vi "System-LoadCalibration.vi"   [LabVIEW 2016, in "DSI-RT.lvlib"]
uses:
  DSI-RT.lvlib
  <vilib>/addons/Software Calibration Management/xSCM/CalPoint-Load Calibration.vi
  <vilib>/addons/Software Calibration Management/xSCM/CalPoint-Calibration File Path.vi
  <vilib>/addons/Software Calibration Management/xSCM/CalPoint-Read Calibration.vi
  <vilib>/addons/Software Calibration Management/xSCM/SubVIs/Recompose Type.vi
  <vilib>/addons/Software Calibration Management/xSCM/SubVIs/Match Element.vi
  <vilib>/addons/Software Calibration Management/xSCM/SubVIs/Variant Type Index.vi
  <vilib>/addons/Software Calibration Management/xSCM/SubVIs/Variant Element By Name.vi
  <vilib>/addons/Software Calibration Management/xSCM/SubVIs/Filter Calibration.vi
  <vilib>/addons/Software Calibration Management/xSCM/SubVIs/Remove Units Text.vi
  <vilib>/addons/Software Calibration Management/xSCM/SubVIs/A2L-Flatten Name.vi
  <vilib>/addons/Software Calibration Management/xSCM/CalPoint-Data.vi
  <vilib>/addons/Software Calibration Management/xSCM/SubVIs/Variant Data Index.vi
  <vilib>/addons/Software Calibration Management/xSCM/CalPoint-Set.vi
  <vilib>/addons/Software Calibration Management/xSCM/Set/Set Variant.vi
  <vilib>/addons/Software Calibration Management/xSCM/CalPoint.xnode
  <vilib>/addons/Software Calibration Management/xSCM/ni_scm.dll
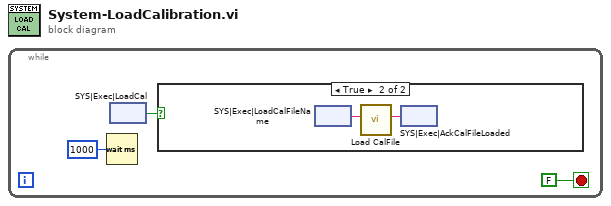
[diagram p0: block diagram]
diagram:
  n1 = while {
    stop <- FALSE stop-if-true
    n2 = Wait (ms)(milliseconds to wait=u32 1000) -> ()  [unwired: 1 out]
    n3 = xnode "SYS|Exec|LoadCal"() -> ("Value"=w1:bool)
    n4 = case shown="True" w1 {
      frame False {
      }
      frame True {
        n5 = xnode "SYS|Exec|LoadCalFileName"() -> ("Value"=w5:string)
        n6 = call <vilib>:"Load CalFile.vi"("LoadCalFileName"=w5) -> ("Ack CalFile Load"=w4:string)  [unwired: 10 in]
        n7 = xnode "SYS|Exec|AckCalFileLoaded"("Value"=w4) -> ()
      }
    }
  }
